vi "Internal Components.vi"(8 "error in (no error)":errorcluster) -> (0 "error out":errorcluster, 3 "Components":refnum<class "Component.lvclass">[](array[class]))   [LabVIEW 2017, in "DSF Core.lvlib"]
uses:
  Component/Component.lvclass
  Component/Component.lvclass/Component.ctl
  Component/Initialize.vi
  Component/Default Buffer Converter/Default Buffer Converter Component.lvclass
  C:/Git/niveristand-data-sharing-framework-custom-device/Core/Classes/Component/Component.lvclass
  Component Configuration/Find.vi
  Component User Interface/Find.vi
  Components/Buffer Converters/DSF Type Converter/Configurations/Default Buffer Converter Configurations.lvclass
  Components/Buffer Converters/DSF Type Converter/User Interfaces/Default Buffer Converter User Interfaces.lvclass
  Components/Buffer Converters/DSF Type Converter/Default Buffer Converter.lvclass
  DSF Core.lvlib
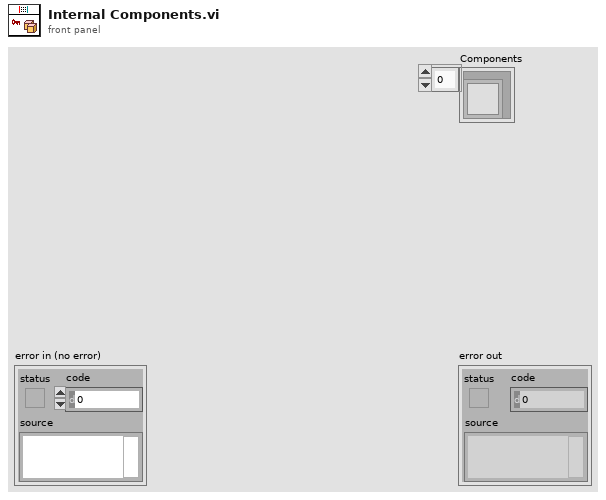
[diagram p1: front panel]
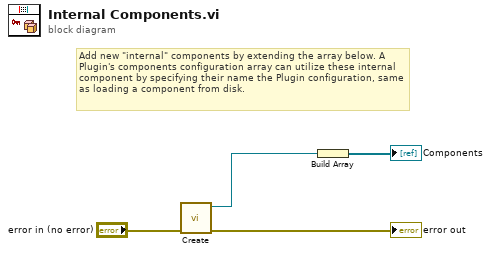
[diagram p0: block diagram]
diagram:
  # "Add new \"internal\" components by extending the array below. A Plugin's components configuration array can utilize these internal component by specifying their name the Plugin configuration, same as loading a component from disk."
  n1 = call "Create.vi"("error in (no error)"="error in (no error)") -> ("error out"=→"error out":errorcluster, "Default Buffer Converter Component"=w1:refnum<class "Default Buffer Converter Component.lvclass">)  [unwired: 9 in]
  n2 = Build Array(w1) -> (→"Components":refnum<class "Default Buffer Converter Component.lvclass">[])
